vi "Jarvis Communication To AI.vi"(8 "Port:":u16=20011, 9 "SSL Vision Address:":string="127.0.0.1") -> ()   [LabVIEW 2017]
uses:
  Varint Encoder uint32.vi
panel:
  in  "Array In":u8[](array[numeric])
  out "error out":errorcluster
  out "Array":u8[](array[numeric]) format="%02x"
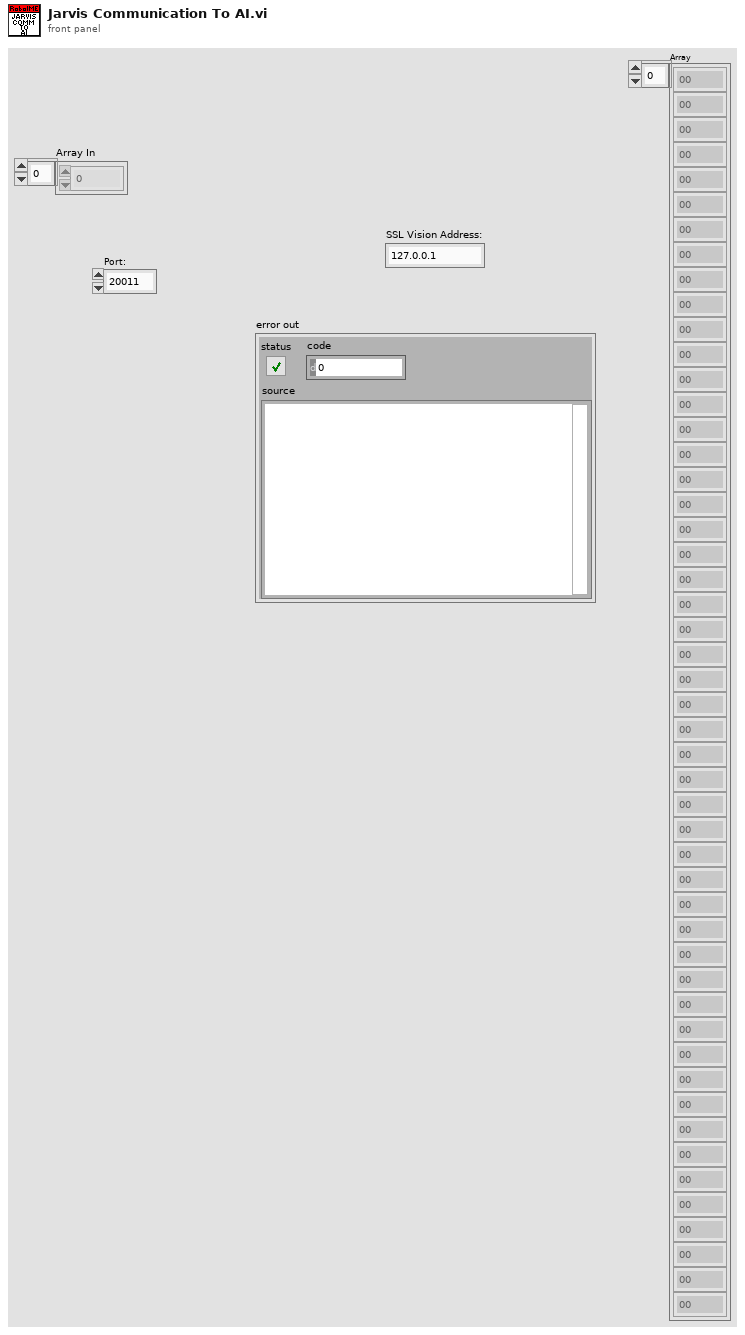
[diagram p1: front panel]
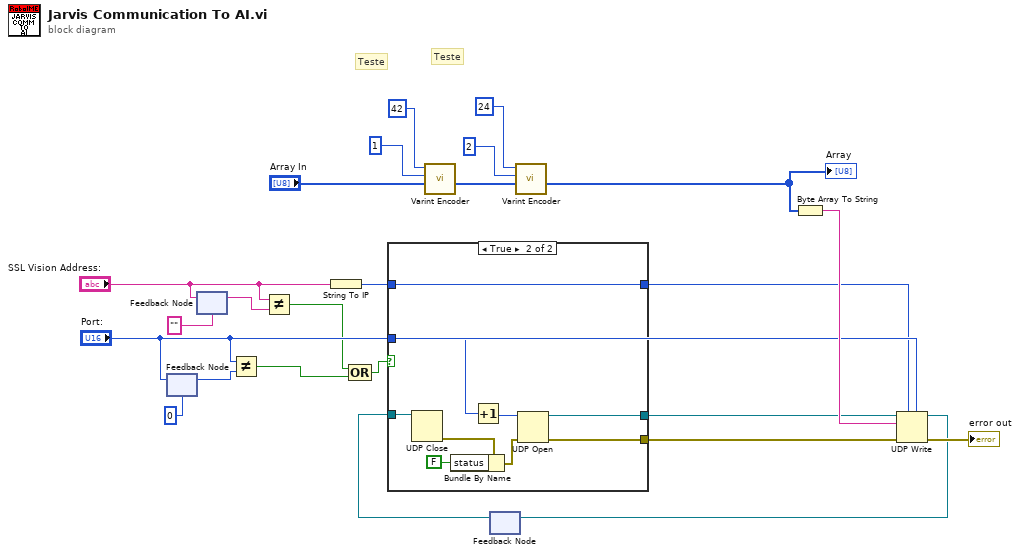
[diagram p0: block diagram]
diagram:
  # "Teste"
  # "Teste"
  n1 = feedback #1(u16 0 ("Port:")) -> (w22:u16)
  n2 = feedback-in #1("Port:") -> ()
  n3 = feedback #2("" ("SSL Vision Address:")) -> (w20:string)
  n4 = feedback-in #2("SSL Vision Address:") -> ()
  n5 = Not Equal?(x="Port:", y=w22) -> (x != y?=w18:bool)
  n6 = Not Equal?(x="SSL Vision Address:", y=w20) -> (x != y?=w19:bool)
  n7 = String To IP(1:"SSL Vision Address:") -> (0:w9:u32)
  n8 = Compound Arithmetic op=OR(w19, w18) -> (w17:bool)
  n9 = call-poly "Varint Encoder.vi"("Array In"="Array In", "Key"=u32 1, "Value"=u32 42) -> ("Array"=w7:u8[])  [unwired: 8 in]
  n10 = feedback #3() -> (w15:refnum<k16>)  [unwired: 1 in]
  n11 = case shown="True" w17 {
    tunnel: [_ w35] -> w23
    tunnel: [w26 w33] -> w14
    tunnel: "Port:" -> [_ w32]
    tunnel: w9 -> [w25 w30]
    tunnel: w15 -> [w26 w31]
    tunnel: [w25 w30] -> w8
    frame False {
    }
    frame True {
      n12 = UDP Close(connection ID=w31) -> (error out=w29:errorcluster)  [unwired: 1 in, 1 out]
      n13 = Bundle By Name(cluster=w29, "status"=FALSE) -> (w28:errorcluster)
      n14 = Increment(x=w32) -> (x+1=w34:u16)
      n15 = UDP Open(8:w28, 11:w34) -> (port=w33:refnum<k16>, 0:w35:errorcluster)  [unwired: 3 in, 1 out]
    }
  }
  n16 = call-poly "Varint Encoder.vi"("Array In"=w7, "Key"=u32 2, "Value"=u32 24) -> ("Array"=w1:u8[])  [unwired: 8 in]
  "Array" <- w1
  n17 = Byte Array To String(unsigned byte array=w1) -> (string=w24:string)
  n18 = UDP Write(address=w8, port or service name="Port:", connection ID=w14, data in=w24, 8:w23) -> (error out=→"error out":errorcluster, 3:w13:refnum<k16>)  [unwired: 1 in]
  n19 = feedback-in #3(w13) -> ()
